vi "Test Executive.vi"(11 "Module Config":T30={"Name"="Test Executive", "Parent Q"=refnum, "Is Child?"=FALSE, "Index"=0, "Dirs"={"Root"=path "C:/MTE", "Config"=path "C:/MTE/Config", "Logs"=path "C:/MTE/Logs", "Reports"=path "C:/ATE/Reports", "App Data"=path "C:/ProgramData/Test Executive"}, "Simulate"=FALSE, "SimCtrl"=refnum}) -> ()   [LabVIEW 2018] (continued)
                    n1107 = List Folder(path=w2440) -> (filenames=w2441:string[], folder names=w2442:string[], error out=w2439:errorcluster)  [unwired: 3 in, 1 out]
                    n1108 = Array Size(array=w2441) -> (size(s)=w2443:i32)
                    n1109 = Array Size(array=w2442) -> (size(s)=w2444:i32)
                    n1110 = case shown="\"Passing\", \"PASS\"" w2449 {
                      tunnel: [_ "FAIL" "PASS" "ERROR" "ABORT"] -> w2448
                      frame "None", Default {
                      }
                      frame "Failing", "FAIL" {
                        (unwired) TRUE
                      }
                      frame "Passing", "PASS" {
                        (unwired) TRUE
                      }
                      frame "ERROR" {
                      }
                      frame "ABORT" {
                        (unwired) TRUE
                      }
                    }
                    n1111 = Format Into String(format string="%08d", w2437) -> (resulting string=w2435:string)  [unwired: 2 in, 1 out]
                    n1112 = Greater Than 0?(x=w2443) -> (x > 0?=w2446:bool)
                    n1113 = Greater Than 0?(x=w2444) -> (x > 0?=w2445:bool)
                    n1114 = local read "Seq Rslt"() -> (w2452:string)
                    n1115 = call <vilib>:"File.Check if File or Folder Exists.vi"("Path"=w2440) -> ("Exists"=w2447:bool)  [unwired: 6 in, 4 out]
                    n1116 = Or(x=w2446, y=w2445) -> (x .or. y?=w2438:bool)
                    n1117 = case shown="True" w2447 {
                      tunnel: w2453 -> [_ w2460]
                      tunnel: w2452 -> [_ w2459]
                      tunnel: w2450 -> [_ w2458]
                      tunnel: w2440 -> [_ w2457]
                      tunnel: w2448 -> [_ w2456]
                      tunnel: w2439 -> [_ _]
                      tunnel: w2438 -> [_ w2455]
                      tunnel: w2435 -> [_ w2454]
                      frame False {
                      }
                      frame True {
                        n1118 = case shown="True" w2455 {
                          tunnel: w2460 -> [_ w2472]
                          tunnel: w2459 -> [_ w2471]
                          tunnel: w2458 -> [_ w2466]
                          tunnel: w2457 -> [w2462 w2467]
                          tunnel: w2456 -> [_ w2470]
                          tunnel: [w2461 _] -> _
                          tunnel: w2454 -> [_ w2463]
                          frame False {
                            # "Folder is empty\nDelete it"
                            n1119 = Delete(path (use dialog)=w2462) -> (error out=w2461:errorcluster)  [unwired: 4 in, 2 out]
                          }
                          frame True {
                            # "Assign Task to Copy Folder"
                            n1120 = call "TestExec.Process Options for Archive UUT Folder.vi"("Sequence"=w2471, "Code"=w2463, "Result"=w2470, "Args"=w2472, "ArchiveDir"=w2466, "UUTDir"=w2467) -> ("Error"=w2468:errorcluster, "SubDirs"=w2464:string[], "New Name"=w2465:string)  [unwired: 2 in, 1 out]
                            n1121 = call "File.ArchiveMover, Assign Task.vi"("SubDirs"=w2464, "Q Name"="ArchiveMover", "error in"=w2468, "New Name"=w2465, "DestDir"=w2466, "Source"=w2467) -> ()  [unwired: 5 in, 1 out]
                          }
                        }
                      }
                    }
                  }
                  frame "ArchiveSummaryUUTData" {
                    n1122 = Unbundle By Name(w2489) -> ("UUT Dir"=w2480:path, "CfgFilePaths.Archive"=w2488:path)
                    n1123 = List Folder(path=w2480) -> (filenames=w2481:string[], folder names=w2482:string[], error out=w2479:errorcluster)  [unwired: 3 in, 1 out]
                    n1124 = Array Size(array=w2481) -> (size(s)=w2483:i32)
                    n1125 = Array Size(array=w2482) -> (size(s)=w2484:i32)
                    n1126 = Greater Than 0?(x=w2483) -> (x > 0?=w2486:bool)
                    n1127 = Greater Than 0?(x=w2484) -> (x > 0?=w2485:bool)
                    n1128 = call <vilib>:"File.Check if File or Folder Exists.vi"("Path"=w2480) -> ("Exists"=w2487:bool)  [unwired: 6 in, 4 out]
                    n1129 = Or(x=w2486, y=w2485) -> (x .or. y?=w2478:bool)
                    n1130 = case shown="True" w2487 {
                      tunnel: w2490 -> [_ w2495]
                      tunnel: w2488 -> [_ w2494]
                      tunnel: w2480 -> [_ w2493]
                      tunnel: w2479 -> [_ _]
                      tunnel: w2478 -> [_ w2492]
                      tunnel: [_ w2491] -> w2477
                      frame False {
                      }
                      frame True {
                        n1131 = case shown="True" w2492 {
                          tunnel: w2495 -> [_ w2511]
                          tunnel: w2494 -> [_ w2510]
                          tunnel: w2493 -> [w2497 w2509]
                          tunnel: [w2496 _] -> _
                          tunnel: [_ w2502] -> w2491
                          frame False {
                            # "Folder is empty\nDelete it"
                            n1132 = Delete(path (use dialog)=w2497) -> (error out=w2496:errorcluster)  [unwired: 4 in, 2 out]
                          }
                          frame True {
                            w2504 = T74 -5200 items=["No Error"=0, "Abort"=-2, "Misc"=-5000, "Fixture Error"=-5100, "File IO - General"=-5200, "FIle IO - Config Error"=-5201, "Instrument - General"=-5300, "Instrument - Serial Com"=-5301, "Instrument - Camera"=-5302, "Instrument - PS"=-5303, "Instrument - Oscilloscope"=-5304, "Instrument - Function Gen"=-5305, "Instrument - Load"=-5306, "Instrument - Meter"=-5307, "Instrument - Power Control"=-5308, "Instrument - Motion"=-5309, "Instrument - RF"=-5310, "System Exe"=-5400, "Image Processing"=-5500, "Communication"=-5600, "Script - Syntax Error"=-6000, "Script - Invalid Name or Param"=-6100, "Script - Timeout"=-6200, "Invalid Data"=-6300, "FW Update Error"=-6500] ("Std Code")
                            n1133 = call "TestExec.Process Options for Archive Summary UUT Folder.vi"("Args"=w2511, "ArchiveDir"=w2510, "UUTDir"=w2509) -> ("Destination Files"=w2505:path[], "Source Files"=w2508:path[], "Destination Path"=w2507:path)  [unwired: 5 in, 1 out]
                            n1134 = call <vilib>:"File.Create Folder if Does Not Exist.vi"("Path"=w2507) -> ("error out"=w2506:errorcluster, "Dup Path"=w2500:path)  [unwired: 8 in, 1 out]
                            n1135 = case shown="No Error" w2506 {
                              selector: w2506 -> [_ w2522]
                              tunnel: w2508 -> [w2515 _]
                              tunnel: w2505 -> [w2514 _]
                              tunnel: w2500 -> [_ _]
                              tunnel: [w2512 w2522] -> w2503
                              frame No Error {
                                n1136 = for {
                                tunnel: w2515 -> [w2521] mode=indexing
                                tunnel: [w2520] -> w2513 mode=indexing
                                tunnel: w2514 -> [w2517] mode=indexing
                                n1137 = Strip Path(path=w2517) -> (stripped path=w2519:path)  [unwired: 1 out]
                                n1138 = call <vilib>:"File.Create Folder if Does Not Exist.vi"("Path"=w2519) -> ("error out"=w2518:errorcluster)  [unwired: 8 in, 2 out]
                                n1139 = Copy(8:w2518, 9:TRUE ("overwrite (F)"), 10:w2517, 11:w2521) -> (0:w2520:errorcluster)  [unwired: 1 in, 2 out]
                                }
                                n1140 = Merge Errors(w2513) -> (w2512:errorcluster)
                              }
                              frame Error {
                              }
                            }
                            n1141 = Format Into String(format string="Error copying result summary files to: \"%s\".", w2500) -> (resulting string=w2499:string)  [unwired: 2 in, 1 out]
                            n1142 = call "Error.Set-Change Error Info.vi"("Std Code"=w2504, "Append Details"=FALSE, "error in"=w2503, "Description"=w2499) -> ("error out"=w2502:errorcluster)  [unwired: 7 in]
                          }
                        }
                      }
                    }
                  }
                  frame "ClientAttribute", "TestSetupAttribute" {
                    # "Cmd_ClientAttribute(Name,Value)"
                    n1143 = Unbundle By Name(w2526) -> ("RptHdr.Test Sequence.Config.Config_Item"=w2534:cluster{"Name":string, "Value":string}[])
                    n1144 = Index Array(array=w2527) -> (element #1=w2532:string, element #2=w2531:string)  [unwired: 2 in]
                    n1145 = call <vilib>:"Q.Enqueue Task.vi"("Top of Q"=TRUE, "Task Name"="Update Result Table", "Q In"=w2528) -> ()  [unwired: 7 in, 2 out]
                    n1146 = Bundle By Name(cluster=cluster{"Name":string, "Value":string} {"Name"="", "Value"=""} ("element"), "Name"=w2532, "Value"=w2531) -> (w2523:cluster{"Name":string, "Value":string})
                    n1147 = Build Array (concatenate)(w2534, w2523) -> (w2533:cluster{"Name":string, "Value":string}[])
                    n1148 = Bundle By Name(cluster=w2526, "RptHdr.Test Sequence.Config.Config_Item"=w2533) -> (w2525:T73)
                  }
                  frame "Comment" {
                    n1149 = Index Array(array=w2536) -> (element=w2539:string)  [unwired: 1 in]
                    n1150 = Unbundle By Name(w2537) -> ("Log"=w2540:refnum<class "Event Notification.lvclass">)
                    n1151 = call <vilib>:"Event Notification.Status Message.vi"("Display"=TRUE, "Log"=FALSE, "Level"=Event_Log.Log_Level."Normal", "Message"=w2539, "Event Notification in"=w2540) -> ()  [unwired: 7 in]
                  }
                  frame "CreateUUTFolder" {
                    n1152 = Unbundle By Name(w2558) -> ("CfgFilePaths.LocalData"=w2566:path)
                    n1153 = local read "SN"() -> (w2543:string)
                    n1154 = local read "Start Time"() -> (w2548:timestamp)
                    n1155 = call "File.Create UUT Dir.vi"("Start Time"=w2548, "SN"=w2543, "Local Data Dir"=w2566) -> ("error out"=w2565:errorcluster, "UUTDir"=w2552:path)  [unwired: 6 in, 1 out]
                    n1156 = Format Date/Time String(time format string (%c)="%Y%m%d_%H%M%S", seconds (now)=w2548) -> (date/time string=w2547:string)  [unwired: 1 in]
                    n1157 = Path To String(path=w2552) -> (string=w2568:string)
                    n1158 = Unbundle By Name(w2558) -> ("StaApp"=w2570:string)
                    n1159 = Build Array("SN", w2543) -> (w2546:string[])
                    n1160 = Build Array("UUTDir", w2568) -> (w2559:string[])
                    n1161 = Build Array("StartTime", w2547) -> (w2545:string[])
                    n1162 = To Variant(anything=w2552) -> (Variant=w2564:variant)
                    n1163 = Unbundle By Name(w2558) -> ("SeqMgr"=w2561:refnum<class "SeqMgr.lvclass">)
                    n1164 = Build Array(w2559, w2546, w2545) -> (w2563:string[][])
                    n1165 = call <vilib>:"Q.Enqueue Task.vi"("Data1"=w2564, "Q Name"=w2570, "Task Name"="Update UUT Folder") -> ()  [unwired: 7 in, 2 out]
                    n1166 = call <vilib>:"SeqMgr.Variables - Add, Replace.vi"("Name, Value"=w2563, "SeqMgr in"=w2561) -> ("SeqMgr out"=w2562:refnum<class "SeqMgr.lvclass">)  [unwired: 8 in, 1 out]
                    n1167 = Bundle By Name(cluster=w2558, "SeqMgr"=w2562, "UUT Dir"=w2552) -> (w2560:T73)
                    n1168 = Unbundle By Name(w2551) -> ("Log"=w2556:refnum<class "Event Notification.lvclass">)
                    n1169 = Format Into String(format string="Create UUT Folder \"%s\"", w2552) -> (resulting string=w2557:string)  [unwired: 2 in, 1 out]
                    n1170 = call <vilib>:"Event Notification.Status Message.vi"("Log"=TRUE, "Level"=Event_Log.Log_Level."Debug1", "Message"=w2557, "Event Notification in"=w2556) -> ()  [unwired: 8 in]
                  }
                  frame "CreateCsvReport" {
                    # "Cmd_CreateCsvReport(Folder)"
                    n1171 = Unbundle By Name(w2581) -> ("RptHdr"=w2589:T70, "RptUUT"=w2605:T50, "Data.Meas"=w2604:T38[], "ResultState"=w2598:T63)
                    n1172 = local read "Comment"() -> (w2582:string)
                    n1173 = Unbundle By Name(w2598) -> ("Code"=w2597:i32, "Description"=w2596:string, "State"=w2595:T1)
                    n1174 = Index Array(array=w2585) -> (element=w2592:string)  [unwired: 1 in]
                    n1175 = case shown="True" "Comment At End" {
                      tunnel: w2582 -> [w2607 w2612]
                      tunnel: [w2607 w2611] -> w2580
                      tunnel: w2581 -> [w2606 w2610]
                      tunnel: [w2606 w2609] -> w2579
                      frame False {
                      }
                      frame True {
                        n1176 = Bundle By Name(cluster=w2610, "Lists.CmtPrmpt"=TRUE) -> (w2609:T73)
                        n1177 = call "TestExec.Prompt for entering Comment.vi"("Comment"=w2612) -> ("Comment Out"=w2611:string)  [unwired: 10 in]
                      }
                    }
                    n1178 = case shown="\"Passing\", \"PASS\"" w2595 {
                      tunnel: [TestResult.Symptom.State."Completed" ("Result.Result") TestResult.Symptom.State."Pass" ("Result.Result") TestResult.Symptom.State."Fail" ("Result.Result") TestResult.Symptom.State."Aborted" ("Result.Result") TestResult.Symptom.State."Error" ("Result.Result")] -> w2594
                      frame "None", Default {
                      }
                      frame "Passing", "PASS" {
                      }
                      frame "Failing", "FAIL" {
                      }
                      frame "ABORT" {
                      }
                      frame "ERROR" {
                      }
                    }
                    n1179 = String To Path(string=w2592) -> (path=w2591:path)
                    n1180 = Bundle By Name(cluster=w2605, "Measurements.Measurement"=w2604, "Result.Code"=w2597, "Result.Description"=w2596, "Result.Result"=w2594) -> (w2600:T50)
                    n1181 = local read "Duration(s)"() -> (w2587:dbl)
                    n1182 = call <vilib>:"File.Check if File or Folder Exists.vi"("Path"=w2591) -> ("Exists"=w2590:bool, "Dup Path"=w2571:path)  [unwired: 6 in, 3 out]
                    n1183 = Bundle By Name(cluster=w2589, "Test Run.Comment"=w2580, "Test Run.Duration(s)"=w2587) -> (w2588:T70)
                    n1184 = Unbundle By Name(w2588) -> ("Station"=w2603:T47, "Test Run"=w2602:T48, "Test Sequence"=w2601:T49)
                    n1185 = Bundle By Name(cluster=w2579, "RptHdr.Test Run.Comment"=w2580) -> (w2578:T73)
                    n1186 = Build Array(w2600) -> (w2599:T50[])
                    n1187 = Bundle By Name(cluster=T46 {"#attributes"={"Version"="MTE_1.0.0"}, "Station"={"Name"="", "PN"="", "SN"="", "Rev"="", "PC Name"="", "Location"="", "HW_Config"={"HW_Item"=[]}, "SW_Config"={"SW_Item"=[]}}, "Test Run"={"Operator"="", "Start Time"=timestamp(0 s since 1904-01-01), "Duration(s)"=0.0, "Mode"="", "Comment"="", "ProcessStep"=""}, "Test Sequence"={"Name"="", "Config"={"Config_Item"=[]}}, "UUTs"={"UUT"=[]}} ("Test Result"), "Station"=w2603, "Test Run"=w2602, "Test Sequence"=w2601, "UUTs.UUT"=w2599) -> (w2593:T46)
                    n1188 = case shown="False" w2590 {
                      tunnel: w2593 -> [_ w2622]
                      tunnel: w2571 -> [w2617 w2620]
                      tunnel: [w2615 w2621] -> w2584
                      frame False {
                        w2616 = T74 -6100 items=["No Error"=0, "Abort"=-2, "Misc"=-5000, "Fixture Error"=-5100, "File IO - General"=-5200, "FIle IO - Config Error"=-5201, "Instrument - General"=-5300, "Instrument - Serial Com"=-5301, "Instrument - Camera"=-5302, "Instrument - PS"=-5303, "Instrument - Oscilloscope"=-5304, "Instrument - Function Gen"=-5305, "Instrument - Load"=-5306, "Instrument - Meter"=-5307, "Instrument - Power Control"=-5308, "Instrument - Motion"=-5309, "Instrument - RF"=-5310, "System Exe"=-5400, "Image Processing"=-5500, "Communication"=-5600, "Script - Syntax Error"=-6000, "Script - Invalid Name or Param"=-6100, "Script - Timeout"=-6200, "Invalid Data"=-6300, "FW Update Error"=-6500] ("Std Code")
                        n1189 = Format Into String(format string="Can not create CSV report.  Dir does not exist: \"%s\"", w2617) -> (resulting string=w2614:string)  [unwired: 2 in, 1 out]
                        n1190 = call "Error.Set-Change Error Info.vi"("Std Code"=w2616, "Description"=w2614, "Set Error"=TRUE) -> ("error out"=w2615:errorcluster)  [unwired: 8 in]
                      }
                      frame True {
                        n1191 = call "Result.Report Creator.vi"("Use UUTFolderName"=TRUE, "Data"=w2622, "Format"=Result.Report_Format_Selector."CSV", "OutputDir"=w2620) -> ("error out"=w2621:errorcluster)  [unwired: 6 in, 1 out]
                      }
                    }
                    n1192 = Unbundle By Name(w2572) -> ("Log"=w2576:refnum<class "Event Notification.lvclass">)
                    n1193 = Format Into String(format string="Create CSV Report in \"%s\"", w2571) -> (resulting string=w2577:string)  [unwired: 2 in, 1 out]
                    n1194 = call <vilib>:"Event Notification.Status Message.vi"("Log"=TRUE, "Level"=Event_Log.Log_Level."Debug1", "Message"=w2577, "Event Notification in"=w2576) -> ()  [unwired: 8 in]
                  }
                  frame "DataPrompt" {
                    # "DataPrompt(PromptText,VarName)"
                    n1195 = while {
                      shift-right: [w2638] -> w2632
                      shift-left: w2633 -> [w2641]
                      shift-right: [w2637] -> _
                      shift-left: "Init" -> [w2642]
                      tunnel: w2631 -> [w2640]
                      tunnel: w2630 -> [w2639]
                      tunnel: [w2635] -> w2629
                      stop <- w2636 stop-if-true
                      n1196 = case shown="\"Done\", Default" w2642 {
                        tunnel: w2641 -> [w2647 w2663 w2677 w2703 w2710 w2714]
                        tunnel: w2640 -> [w2643 w2660 _ w2701 _ _]
                        tunnel: w2639 -> [w2645 _ _ _ _ w2717]
                        tunnel: [w2647 w2663 w2677 w2704 w2710 w2714] -> w2638
                        tunnel: [w2646 "Wait on Input" "Read Data" "Disable Controls" "Done" _] -> w2637
                        tunnel: [_ _ _ _ _ TRUE] -> w2636
                        tunnel: [w2644 _ _ _ _ w2717] -> w2635
                        frame "Init" {
                          n1197 = case shown="No Error" w2645 {
                            selector: w2645 -> [_ w2655]
                            tunnel: ["Enable Controls" "Done"] -> w2646
                            tunnel: [_ w2655] -> w2644
                            tunnel: w2643 -> [w2650 _]
                            frame No Error {
                              w2648 = T6."Prompt" ("Test Status Tab")
                              n1198 = Index Array(array=w2650) -> (element=→"OperPrompt2":string)  [unwired: 1 in]
                              n1199 = local write "Test Status Tab"(w2648) -> ()
                              n1200 = local write "Test Status Tab Sel"(w2648) -> ()
                              n1201 = property on="Status" class="Str"("Text.Text"="Waiting for Operator input on Prompt page.", "Text.BGColor"=u32 16774001, "Blinking"=TRUE) -> ()  [unwired: 2 in, 2 out]
                            }
                            frame Error {
                            }
                          }
                        }
                        frame "Enable Controls" {
                          w2661 = T36."Enabled" ("Disabled")
                          n1202 = Index Array(array=w2660, index=2) -> (element=w2657:string)
                          n1203 = property on="Prompt2_OK" class="Bool"("DisabledEnum"=w2661) -> ()  [unwired: 2 in, 2 out]
                          n1204 = property on="Prompt YES" class="Bool"("DisabledEnum"=w2661) -> ()  [unwired: 2 in, 2 out]
                          n1205 = property on="Prompt NO" class="Bool"("DisabledEnum"=w2661) -> ()  [unwired: 2 in, 2 out]
                          n1206 = property on="OperInput Data" class="Str"("DisabledEnum"=w2661) -> (error out=w2658:errorcluster)  [unwired: 2 in, 1 out]
                          n1207 = case shown="\"\", \"0\", Default" w2657 {
                            tunnel: w2658 -> [_ _ _]
                            frame "", "0", Default {
                              w2665 = FALSE ("Visible")
                              n1208 = property on="Prompt2_OK" class="Bool"("Visible"=TRUE) -> ()  [unwired: 2 in, 2 out]
                              n1209 = property on="OperInput Data" class="Str"("Visible"=TRUE ("Key Focus")) -> ()  [unwired: 2 in, 2 out]
                              n1210 = property on="Prompt YES" class="Bool"("Visible"=w2665) -> ()  [unwired: 2 in, 2 out]
                              n1211 = property on="Prompt NO" class="Bool"("Visible"=w2665) -> ()  [unwired: 2 in, 2 out]
                              n1212 = property on="OperInput Data" class="Str"("Key Focus"=TRUE) -> ()  [unwired: 2 in, 2 out]
                            }
                            frame "1" {
                              w2670 = FALSE ("Visible")
                              n1213 = property on="OperInput Data" class="Str"("Visible"=FALSE) -> ()  [unwired: 2 in, 2 out]
                              n1214 = property on="Prompt YES" class="Bool"("Visible"=w2670) -> ()  [unwired: 2 in, 2 out]
                              n1215 = property on="Prompt NO" class="Bool"("Visible"=w2670) -> ()  [unwired: 2 in, 2 out]
                              n1216 = property on="Prompt2_OK" class="Bool"("Key Focus"=TRUE) -> ()  [unwired: 2 in, 2 out]
                              n1217 = property on="Prompt2_OK" class="Bool"("Visible"=TRUE ("Key Focus")) -> ()  [unwired: 2 in, 2 out]
                            }
                            frame "2" {
                              w2673 = TRUE ("Visible")
                              n1218 = property on="OperInput Data" class="Str"("Visible"=FALSE) -> ()  [unwired: 2 in, 2 out]
                              n1219 = property on="Prompt2_OK" class="Bool"("Visible"=FALSE ("Key Focus")) -> ()  [unwired: 2 in, 2 out]
                              n1220 = property on="Prompt YES" class="Bool"("Visible"=w2673) -> ()  [unwired: 2 in, 2 out]
                              n1221 = property on="Prompt NO" class="Bool"("Visible"=w2673) -> ()  [unwired: 2 in, 2 out]
                              n1222 = property on="Prompt YES" class="Bool"("Key Focus"=TRUE ("Visible")) -> ()  [unwired: 2 in, 2 out]
                            }
                          }
                        }
                        frame "Wait on Input" {
                          n1223 = while {
                            stop <- w2678 stop-if-true
                            n1224 = event shown="[1] \"Prompt2_OK\": Value Change" {
                              selector: _ -> [_ _ _ _]
                              dyn-events: _ -> [_ _ _ _]
                              timeout: 100 -> [_ _ _ _]
                              tunnel: [w2680 TRUE TRUE TRUE] -> w2678
                              event Timeout {
                                n1225 = event-data() -> ()  [unwired: 1 in, 3 out]
                                n1226 = local read "Abort Flag"() -> (w2680:bool)
                              }
                              event "Prompt2_OK": Value Change {
                                n1227 = event-data() -> ()  [unwired: 1 in, 6 out]
                              }
                              event "Prompt YES", "Prompt NO": Value Change {
                                n1228 = event-data() -> ()  [unwired: 1 in, 6 out]
                                n1229 = Select(t="YES", s="Prompt YES", f="NO") -> (s? t:f=w2683:string)
                                n1230 = local write "OperInput Data"(w2683) -> ()
                              }
                              event "OperInput Data": Value Change {
                                n1231 = event-data() -> ()  [unwired: 1 in, 6 out]
                              }
                            }
                          }
                        }
                        frame "Read Data" {
                          n1232 = Index Array(array=w2701, index=1) -> (element=w2697:string)
                          n1233 = call <vilib>:"Trim Whitespace.vi"("string"=w2697) -> ("trimmed string"=w2696:string)  [unwired: 1 in]
                          n1234 = call <vilib>:"Trim Whitespace.vi"("string"="OperInput Data") -> ("trimmed string"=w2688:string)  [unwired: 1 in]
                          n1235 = Empty String/Path?(string/path=w2696) -> (empty?=w2699:bool)
                          n1236 = Select(t="OperatorDataInput", s=w2699, f=w2696) -> (s? t:f=w2694:string)
                          n1237 = Build Array(w2694, w2688) -> (w2695:string[])
                          n1238 = Unbundle By Name(w2703) -> ("SeqMgr"=w2706:refnum<class "SeqMgr.lvclass">)
                          n1239 = Build Array(w2695) -> (w2702:string[][])
                          n1240 = Format Into String(format string="Input data = %s", w2688) -> (resulting string=w2692:string)  [unwired: 2 in, 1 out]
                          n1241 = call <vilib>:"SeqMgr.Variables - Add, Replace.vi"("Name, Value"=w2702, "SeqMgr in"=w2706) -> ("SeqMgr out"=w2705:refnum<class "SeqMgr.lvclass">)  [unwired: 8 in, 1 out]
                          n1242 = Bundle By Name(cluster=w2703, "SeqMgr"=w2705) -> (w2704:T73)
                          n1243 = property on="Status" class="Str"("Text.Text"=w2692, "Text.BGColor"=u32 16448250, "Blinking"=FALSE) -> ()  [unwired: 2 in, 2 out]
                        }
                        frame "Disable Controls" {
                          w2708 = T36."Disabled and Grayed Out" ("Disabled")
                          n1244 = property on="Prompt2_OK" class="Bool"("DisabledEnum"=w2708) -> ()  [unwired: 2 in, 2 out]
                          n1245 = property on="Prompt YES" class="Bool"("DisabledEnum"=w2708) -> ()  [unwired: 2 in, 2 out]
                          n1246 = property on="Prompt NO" class="Bool"("DisabledEnum"=w2708) -> ()  [unwired: 2 in, 2 out]
                          n1247 = property on="OperInput Data" class="Str"("DisabledEnum"=w2708) -> ()  [unwired: 2 in, 2 out]
                        }
                        frame "Done", Default {
                          n1248 = Unbundle By Name(w2714) -> ("Opts.DispDetails"=w2715:bool)
                          n1249 = invoke on="OperPrompt2" class="Str" method="Reinit To Default"() -> ()  [unwired: 3 in, 3 out]
                          n1250 = invoke on="OperInput Data" class="Str" method="Reinit To Default"() -> ()  [unwired: 3 in, 3 out]
                          n1251 = Select(t=1, s=w2715, f=0) -> (s? t:f=w2711:i32)
                          n1252 = property on="Prompt2_OK" class="Bool"("DisabledEnum"=T36."Disabled and Grayed Out" ("Disabled")) -> ()  [unwired: 2 in, 2 out]
                          n1253 = local write "Test Status Tab Sel"(w2711) -> ()
                          n1254 = local write "Test Status Tab"(w2711) -> ()
                        }
                      }
                    }
                  }
                  frame "Delay", "Wait" {
                    # "Wait(Secs)"
                    n1255 = Unbundle By Name(w2731) -> ("Log"=w2720:refnum<class "Event Notification.lvclass">)
                    n1256 = local read "Status"() -> (w2728:string)
                    n1257 = Index Array(array=w2719) -> (element=w2729:string)  [unwired: 1 in]
                    n1258 = Concatenate Strings(w2728, "\r\n") -> (w2727:string)
                    n1259 = Fract/Exp String To Number(string=w2729) -> (number=w2726:dbl)  [unwired: 3 in, 1 out]
                    n1260 = Format Into String(format string="Delaying for %s seconds.", initial string=w2727, w2729) -> (resulting string=w2725:string)  [unwired: 1 in, 1 out]
                    n1261 = call <vilib>:"Event Notification.Status Message.vi"("Log"=FALSE, "Level"=Event_Log.Log_Level."Normal", "Message"=w2725, "Event Notification in"=w2720) -> ()  [unwired: 8 in]
                    n1262 = call <vilib>:"High Resolution Relative Seconds.vi"() -> ("relative seconds"=w2730:dbl)
                    n1263 = while {
                      tunnel: w2730 -> [w2745]
                      tunnel: w2726 -> [w2739]
                      stop <- w2743 stop-if-true
                      # "Remain"
                      # "Elapsed"
                      n1264 = call <vilib>:"High Resolution Relative Seconds.vi"() -> ("relative seconds"=w2746:dbl)
                      n1265 = Subtract(x=w2746, y=w2745) -> (x-y=w2738:dbl)
                      n1266 = Subtract(x=w2739, y=w2738) -> (x-y=w2736:dbl)
                      n1267 = local read "Status"() -> (w2742:string)
                      n1268 = Less Or Equal To 0?(x=w2736) -> (x <= 0?=w2737:bool)
                      n1269 = Multiply(x=w2736, y=1000.0) -> (x*y=w2733:dbl)
                      n1270 = local read "Abort Flag"() -> (w2744:bool)
                      n1271 = Concatenate Strings(w2742, " .") -> (w2740:string)
                      n1272 = To Unsigned Long Integer(number=w2733) -> (unsigned 32bit integer=w2734:u32)
                      n1273 = local write "Status"(w2740) -> ()
                      n1274 = case shown="False" w2737 {
                        tunnel: w2734 -> [w2750 _]
                        frame False {
                          n1275 = In Range and Coerce(upper limit=u32 500 ("lower limit"), x=w2750, lower limit=u32 10) -> (coerced(x)=w2747:u32)  [unwired: 1 out]
                          n1276 = Wait (ms)(milliseconds to wait=w2747) -> ()  [unwired: 1 out]
                        }
                        frame True {
                        }
                      }
                      n1277 = Or(x=w2737, y=w2744) -> (x .or. y?=w2743:bool)
                    }
                  }
                  frame "DeviceEnumCheck" {
                    # "EnumCheck(VID,PID,[RtnVarName])"
                    n1278 = Index Array(array=w2756) -> (element #1=w2755:string, element #2=w2754:string, element #3=w2760:string)  [unwired: 3 in]
                    n1279 = case shown="\"\"" w2760 {
                      selector: w2760 -> [w2783 _]
                      tunnel: [w2783 "DeviceIsEnumerated"] -> w2759
                      frame Default {
                      }
                      frame "" {
                      }
                    }
                    n1280 = Empty String/Path?(string/path=w2755) -> (empty?=w2753:bool)
                    n1281 = Empty String/Path?(string/path=w2754) -> (empty?=w2752:bool)
                    n1282 = And(x=w2753, y=w2752) -> (x .and. y?=w2751:bool)
                    n1283 = case shown="True" w2751 {
                      tunnel: w2759 -> [w2768 _]
                      tunnel: w2758 -> [w2766 w2778]
                      tunnel: [w2765 w2776] -> w2757
                      tunnel: w2755 -> [w2762 _]
                      tunnel: w2754 -> [w2761 _]
                      frame False {
                        n1284 = call "USB.Check Device using PID and VID.vi"("PID"=w2761, "VID"=w2762) -> ("error out"=w2763:errorcluster, "Found"=w2764:bool)  [unwired: 6 in, 2 out]
                        n1285 = call <vilib>:"Clear Errors.vi"("error in (no error)"=w2763) -> ()  [unwired: 5 in, 2 out]
                        n1286 = Select(t="1", s=w2764, f="0") -> (s? t:f=w2770:string)
                        n1287 = Build Array(w2768, w2770) -> (w2769:string[])
                        n1288 = Unbundle By Name(w2766) -> ("SeqMgr"=w2774:refnum<class "SeqMgr.lvclass">)
                        n1289 = Build Array(w2769) -> (w2767:string[][])
                        n1290 = call <vilib>:"SeqMgr.Variables - Add, Replace.vi"("Name, Value"=w2767, "SeqMgr in"=w2774) -> ("SeqMgr out"=w2773:refnum<class "SeqMgr.lvclass">)  [unwired: 8 in, 1 out]
                        n1291 = Bundle By Name(cluster=w2766, "SeqMgr"=w2773) -> (w2765:T73)
                      }
                      frame True {
                        w2775 = T74 -6100 items=["No Error"=0, "Abort"=-2, "Misc"=-5000, "Fixture Error"=-5100, "File IO - General"=-5200, "FIle IO - Config Error"=-5201, "Instrument - General"=-5300, "Instrument - Serial Com"=-5301, "Instrument - Camera"=-5302, "Instrument - PS"=-5303, "Instrument - Oscilloscope"=-5304, "Instrument - Function Gen"=-5305, "Instrument - Load"=-5306, "Instrument - Meter"=-5307, "Instrument - Power Control"=-5308, "Instrument - Motion"=-5309, "Instrument - RF"=-5310, "System Exe"=-5400, "Image Processing"=-5500, "Communication"=-5600, "Script - Syntax Error"=-6000, "Script - Invalid Name or Param"=-6100, "Script - Timeout"=-6200, "Invalid Data"=-6300, "FW Update Error"=-6500] ("Code")
                        n1292 = Unbundle By Name(w2778) -> ("Lists.Limits"=w2782:variant, "ResultState"=w2781:T63)
                        n1293 = call "TestExec.Set Result State.vi"("Code Enum"=w2775, "Limits"=w2782, "Description"="DeviceEnumCheck Error, both VID and PID arguements cannot be empty.", "State"=SeqMgr.Result_State_Enum."ERROR", "Result State In"=w2781) -> ("Result State Out"=w2777:T63)  [unwired: 6 in]
                        n1294 = Bundle By Name(cluster=w2778, "ResultState"=w2777) -> (w2776:T73)
                      }
                    }
                  }
                  frame "Devcon_ListDevices", "Devcon_RemoveDevice", "Devcon_RemoveDevices", "Devcon_Rescan" {
                    n1295 = Unbundle By Name(w2788) -> ("CfgFilePaths.Devcon"=w2791:path)
                    n1296 = case shown="\"Devcon_RemoveDevices\"" w2793 {
                      tunnel: w2792 -> [_ w2806 w2823 w2844 _]
                      tunnel: w2791 -> [_ w2807 w2824 w2845 w2860]
                      tunnel: [_ w2795 w2821 w2838 w2852] -> w2786
                      tunnel: [_ w2794 w2814 w2828 w2853] -> w2785
                      frame Default {
                      }
                      frame "Devcon_ListDevices" {
                        n1297 = Index Array(array=w2806) -> (element #1=w2805:string, element #2=w2804:string)  [unwired: 2 in]
                        n1298 = Equal?(x=w2804, y="1") -> (x = y?=w2802:bool)
                        n1299 = call "Devcon.Find Devices.vi"("State(Present(F), All(T))"=w2802, "DeviceID"=w2805, "DevconEXE"=w2807) -> ("error out"=w2794:errorcluster, "Device List"=w2798:string[][], "Device Cnt"=w2800:i32)  [unwired: 4 in, 2 out]
                        n1300 = for {
                          tunnel: w2798 -> [w2813] mode=indexing
                          tunnel: [w2808] -> w2796 mode=indexing
                          i -> [w2811]
                          n1301 = Index Array(array=w2813) -> (element=w2809:string)  [unwired: 1 in]
                          n1302 = Format Into String(format string="Device_%d", w2811) -> (resulting string=w2810:string)  [unwired: 2 in, 1 out]
                          n1303 = Build Array(w2810, w2809) -> (w2808:string[])
                        }
                        n1304 = Number To Decimal String(number=w2800) -> (decimal integer string=w2799:string)  [unwired: 1 in]
                        n1305 = Build Array("DeviceCount", w2799) -> (w2797:string[])
                        n1306 = Build Array (concatenate)(w2797, w2796) -> (w2795:string[][])
                      }
                      frame "Devcon_RemoveDevice" {
                        n1307 = Index Array(array=w2823) -> (element #1=w2822:string)  [unwired: 2 in, 1 out]
                        n1308 = call "Devcon.Remove Device.vi"("DeviceID"=w2822, "DevconEXE"=w2824) -> ("error out"=w2814:errorcluster, "Success"=w2817:bool)  [unwired: 6 in, 2 out]
                        n1309 = Select(t="1", s=w2817, f="0") -> (s? t:f=w2819:string)
                        n1310 = Build Array("DeviceRemoveSuccess", w2819) -> (w2816:string[])
                        n1311 = Build Array(w2816) -> (w2821:string[][])
                      }
                      frame "Devcon_RemoveDevices" {
                        n1312 = Index Array(array=w2844) -> (element #1=w2843:string, element #2=w2826:string)  [unwired: 2 in]
                        n1313 = Equal?(x=w2826, y="1") -> (x = y?=w2825:bool)
                        n1314 = call "Devcon.Remove Devices.vi"("State(Present(F), All(T))"=w2825, "DeviceID"=w2843, "DevconEXE"=w2845) -> ("error out"=w2828:errorcluster, "Success"=w2833:bool, "Device List"=w2836:string[][])  [unwired: 4 in, 2 out]
                        n1315 = Array Size(array=w2836) -> (size(s)=w2837:i32[])
                        n1316 = Index Array(array=w2837) -> (element=w2835:i32)  [unwired: 1 in]
                        n1317 = for {
                          tunnel: w2836 -> [w2851] mode=indexing
                          tunnel: [w2846] -> w2839 mode=indexing
                          i -> [w2849]
                          n1318 = Index Array(array=w2851) -> (element=w2847:string)  [unwired: 1 in]
                          n1319 = Format Into String(format string="Device_%d", w2849) -> (resulting string=w2848:string)  [unwired: 2 in, 1 out]
                          n1320 = Build Array(w2848, w2847) -> (w2846:string[])
                        }
                        n1321 = Select(t="1", s=w2833, f="0") -> (s? t:f=w2831:string)
                        n1322 = Number To Decimal String(number=w2835) -> (decimal integer string=w2841:string)  [unwired: 1 in]
                        n1323 = Build Array("DeviceCount", w2841) -> (w2840:string[])
                        n1324 = Build Array("DeviceRemoveSuccess", w2831) -> (w2829:string[])
                        n1325 = Build Array (concatenate)(w2840, w2839, w2829) -> (w2838:string[][])
                      }
                      frame "Devcon_Rescan" {
                        n1326 = call "Devcon.Rescan for New Devices.vi"("DevconEXE"=w2860) -> ("error out"=w2853:errorcluster, "Success"=w2854:bool)  [unwired: 9 in]
                        n1327 = Select(t="1", s=w2854, f="0") -> (s? t:f=w2858:string)
                        n1328 = Build Array("DeviceRescanSuccess", w2858) -> (w2856:string[])
                        n1329 = Build Array(w2856) -> (w2852:string[][])
                      }
                    }
                    n1330 = Unbundle By Name(w2788) -> ("SeqMgr"=w2790:refnum<class "SeqMgr.lvclass">)
                    n1331 = call <vilib>:"SeqMgr.Variables - Add, Replace.vi"("Name, Value"=w2786, "SeqMgr in"=w2790) -> ("SeqMgr out"=w2789:refnum<class "SeqMgr.lvclass">)  [unwired: 8 in, 1 out]
                    n1332 = Bundle By Name(cluster=w2788, "SeqMgr"=w2789) -> (w2787:T73)
                  }
                  frame "Error", "SetError" {
                    # "SetError(Code, Desc)"
                    n1333 = Index Array(array=w2873) -> (element #1=w2862:string, element #2=w2866:string)  [unwired: 2 in]
                    n1334 = Unbundle By Name(w2871) -> ("Lists.Limits"=w2878:variant)
                    n1335 = Decimal String To Number(string=w2862) -> (number=w2864:i32)  [unwired: 2 in, 1 out]
                    n1336 = Get Variant Attribute(Variant=w2878, name="CodePrefix", default value (empty Variant)=T25 {"Name"="", "LimType"=enum."None", "LL"="", "UL"="", "Units"="", "FailCode"=0, "FailDesc"=""} ("Result.Test Limit Item")) -> (value=w2880:T25)  [unwired: 1 in, 3 out]
                    n1337 = Equal To 0?(x=w2864) -> (x = 0?=w2865:bool)
                    n1338 = Unbundle By Name(w2880) -> ("FailCode"=w2876:i32)
                    n1339 = Select(t=-5000, s=w2865, f=w2864) -> (s? t:f=w2861:i32)
                    n1340 = call <vilib>:"Q.Enqueue Task.vi"("Top of Q"=TRUE, "Task Name"="Sta Test Status", "Q In"=w2868) -> ()  [unwired: 7 in, 2 out]
                    n1341 = call "TestExec.Append Fault Code Prefix.vi"("Positive(F)\\Negative(T)"=TRUE ("Positive(F)\\Negative(T)"), "FaultCode"=w2861, "FaultCode Prefix"=w2876) -> ("New Fault Code"=w2875:i32)  [unwired: 8 in]
                    n1342 = Bundle By Name(cluster=w2871, "ResultState.State"=SeqMgr.Result_State_Enum."ERROR" ("State"), "ResultState.Code"=w2875, "ResultState.Description"=w2866) -> (w2874:T73)
                    n1343 = Format Into String(format string="Error set by sequence: %s", w2866) -> (resulting string=w2867:string)  [unwired: 2 in, 1 out]
                    n1344 = Unbundle By Name(w2874) -> ("SeqMgr"=w2890:refnum<class "SeqMgr.lvclass">)
                    n1345 = Unbundle By Name(w2872) -> ("Log"=w2884:refnum<class "Event Notification.lvclass">)
                    n1346 = call <vilib>:"SeqMgr.Variables - Add, Replace.vi"("Name, Value"=string[][] [["Error", "1"]] ("appended array"), "SeqMgr in"=w2890) -> ("SeqMgr out"=w2889:refnum<class "SeqMgr.lvclass">)  [unwired: 8 in, 1 out]
                    n1347 = Bundle By Name(cluster=w2874, "SeqMgr"=w2889) -> (w2887:T73)
                    n1348 = call <vilib>:"Event Notification.Status Message.vi"("Log"=TRUE, "Level"=Event_Log.Log_Level."Verbose", "Message"=w2867, "Event Notification in"=w2884) -> ()  [unwired: 8 in]
                  }
                  frame "ImagePrompt" {
                    # "ImagePrompt(PromptMessage,ImageFileFolder,ImageFileName,[ResultAttributeName])"
                    n1349 = while {
                      shift-right: [w2907] -> w2896
                      shift-left: w2897 -> [w2908]
                      tunnel: w2895 -> [_]
                      shift-right: [w2900] -> _
                      shift-left: "Init" -> [w2909]
                      shift-right: [w2901] -> _
                      shift-left: w2893 -> [w2905]
                      shift-right: [w2903] -> _
                      shift-left: _ -> [w2904]
                      tunnel: w2892 -> [w2902]
                      tunnel: w2891 -> [w2898]
                      stop <- w2906 stop-if-true
                      n1350 = case shown="\"Load Image\"" w2909 {
                        tunnel: w2908 -> [w2932 w2952 w2960 w3014]
                        tunnel: [w2932 w2952 w2960 w3014] -> w2907
                        tunnel: ["Load Image" "Get Input" "Done" "Done"] -> w2899
                        tunnel: [_ _ _ TRUE] -> w2906
                        tunnel: w2905 -> [_ _ _ w3001]
                        tunnel: [w2914 w2948 w2954 w3001] -> w2901
                        tunnel: w2904 -> [_ w2947 w2959 w2999]
                        tunnel: [w2923 w2947 w2958 w2999] -> w2903
                        tunnel: w2902 -> [w2928 _ _ _]
                        tunnel: w2898 -> [_ _ _ w2996]
                        frame "Init" {
                          w2919 = FALSE  # OK
                          w2920 = FALSE  # Timeout
                          w2929 = path ""  # Image
                          w2930 = ""  # Name
                          w2912 = T36."Enabled" ("Disabled")
                          n1351 = Index Array(array=w2928) -> (element #1=→"OperPrompt":string, element #2=w2922:string, element #3=w2921:string, element #4=w2926:string)  [unwired: 4 in]
                          n1352 = call "TestExec.Script Function Params to Path.vi"("File"=w2921, "Folder"=w2922) -> ("error out"=w2913:errorcluster, "Exists"=w2917:bool, "Path"=w2915:path)  [unwired: 7 in]
                          n1353 = case shown="\"\"" w2926 {
                            selector: w2926 -> [w2940 _]
                            tunnel: [w2940 "Operator Image Prompt"] -> w2925
                            frame Default {
                            }
                            frame "" {
                            }
                          }
                          n1354 = Not(x=w2917) -> (.not. x?=w2916:bool)
                          n1355 = Or(x=w2916, y=w2913) -> (x .or. y?=w2918:bool)
                          n1356 = case shown="True" w2918 {
                            tunnel: w2915 -> [_ w2934]
                            tunnel: [_ w2933] -> w2914
                            frame False {
                            }
                            frame True {
                              w2939 = T74 -5200 items=["No Error"=0, "Abort"=-2, "Misc"=-5000, "Fixture Error"=-5100, "File IO - General"=-5200, "FIle IO - Config Error"=-5201, "Instrument - General"=-5300, "Instrument - Serial Com"=-5301, "Instrument - Camera"=-5302, "Instrument - PS"=-5303, "Instrument - Oscilloscope"=-5304, "Instrument - Function Gen"=-5305, "Instrument - Load"=-5306, "Instrument - Meter"=-5307, "Instrument - Power Control"=-5308, "Instrument - Motion"=-5309, "Instrument - RF"=-5310, "System Exe"=-5400, "Image Processing"=-5500, "Communication"=-5600, "Script - Syntax Error"=-6000, "Script - Invalid Name or Param"=-6100, "Script - Timeout"=-6200, "Invalid Data"=-6300, "FW Update Error"=-6500] ("Std Code")
                              n1357 = Path To String(path=w2934) -> (string=w2937:string)
                              n1358 = Format Into String(format string="Image file does not exist: \"%s\".", w2937) -> (resulting string=w2936:string)  [unwired: 2 in, 1 out]
                              n1359 = call "Error.Set-Change Error Info.vi"("Std Code"=w2939, "Description"=w2936, "Set Error"=TRUE) -> ("error out"=w2933:errorcluster)  [unwired: 8 in]
                            }
                          }
                          n1360 = Bundle("Name"=w2930, "Image"=w2929, "Timeout"=w2920, "OK"=w2919) -> (w2924:T79)  [unwired: 1 in]
                          n1361 = Bundle By Name(cluster=w2924, "Name"=w2925, "Image"=w2915) -> (w2923:T79)
                          n1362 = invoke on="OperPict" class="Pict" method="Reinit To Default"() -> ()  [unwired: 3 in, 3 out]
                          n1363 = property on="Open Image File" class="Bool"("DisabledEnum"=w2912) -> ()  [unwired: 2 in, 2 out]
                          n1364 = property on="OperNo" class="Bool"("DisabledEnum"=w2912) -> ()  [unwired: 2 in, 2 out]
                          n1365 = property on="OperOK" class="Bool"("DisabledEnum"=w2912) -> ()  [unwired: 2 in, 2 out]
                        }
                        frame "Load Image" {
                          n1366 = Unbundle By Name(w2947) -> ("Image"=w2946:path)
                          "Image Path" <- w2946
                          n1367 = control-ref of="OperPict"() -> (w2950:refnum<vi>)
                          n1368 = call <vilib>:"Graphics.Read Image File and Auto Scale for 2D Picture.vi"("2D Pict Ref"=w2950, "File"=w2946) -> ("error out"=w2948:errorcluster, "Zoom Factor"=w2942:dbl, "2D Pict"=→"OperPict":picture)  [unwired: 7 in]
                          n1369 = property on="Status" class="Str"("Text.Text"="Waiting for Operator input on Image page.", "Text.BGColor"=u32 16774001, "Blinking"=TRUE) -> ()  [unwired: 2 in, 2 out]
                          n1370 = local write "Zoom Img"(w2942) -> ()
                        }
                        frame "Get Input" {
                          w2953 = T6."Image1" ("Test Status Tab")
                          w2963 = 300.0
                          n1371 = property on="OperOK" class="Bool"("Key Focus"=TRUE) -> ()  [unwired: 2 in, 2 out]
                          n1372 = Multiply(x=w2963, y=1000.0) -> (x*y=w2965:dbl)
                          n1373 = Tick Count (ms)() -> (millisecond timer value=w2962:u32)
                          n1374 = To Unsigned Long Integer(number=w2965) -> (unsigned 32bit integer=w2961:u32)
                          n1375 = while {
                            tunnel: w2962 -> [w2981]
                            tunnel: [w2975] -> w2955
                            tunnel: ["OperOK"] -> w2956
                            tunnel: w2961 -> [w2970]
                            stop <- w2983 stop-if-true
                            # "Wait for input"
                            n1376 = Tick Count (ms)() -> (millisecond timer value=w2982:u32)
                            n1377 = local read "Abort Flag"() -> (w2984:bool)
                            n1378 = Subtract(x=w2982, y=w2981) -> (x-y=w2969:u32)
                            n1379 = Subtract(x=w2970, y=w2969) -> (x-y=w2968:u32)
                            n1380 = Greater?(x=w2969, y=w2970) -> (0:w2976:bool)
                            n1381 = And(x=w2976, y="TO_En") -> (x .and. y?=w2975:bool)
                            n1382 = To Double Precision Float(number=w2968) -> (double precision float=w2979:dbl)
                            n1383 = Wait (ms)(milliseconds to wait=u32 100) -> ()  [unwired: 1 out]
                            n1384 = Divide(x=w2979, y=1000.0) -> (x/y=w2972:dbl)
                            n1385 = Greater Or Equal To 0?(x=w2972) -> (x >= 0?=w2973:bool)
                            n1386 = Compound Arithmetic op=OR(w2975, "OperOK", "OperNo", w2984) -> (w2983:bool)
                            n1387 = Select(t=w2972, s=w2973, f=0.0) -> (s? t:f=w2974:dbl)
                            n1388 = local write "OperCntDwn"(w2974) -> ()
                          }
                          n1389 = local write "Test Status Tab"(w2953) -> ()
                          n1390 = local write "Test Status Tab Sel"(w2953) -> ()
                          n1391 = case shown="False" w2955 {
                            tunnel: [_ errorcluster {"status"=TRUE, "code"=-2, "source"="Operator did not respond to image inspection prompt within timeout interval."} ("error constant")] -> w2954
                            frame False {
                            }
                            frame True {
                            }
                          }
                          n1392 = Bundle By Name(cluster=w2959, "Timeout"=w2955, "OK"=w2956) -> (w2958:T79)
                          "OperCntDwn" <- w2963
                        }
                        frame "Done", Default {
                          w2988 = T36."Disabled and Grayed Out" ("Disabled")
                          n1393 = Unbundle By Name(w2999) -> ("OK"=w3000:bool)
                          n1394 = Unbundle By Name(w2999) -> ("Name"=w2998:string)
                          n1395 = Unbundle By Name(w3014) -> ("Opts.DispDetails"=w3012:bool)
                          n1396 = Not(x=w3000) -> (.not. x?=w2990:bool)
                          n1397 = Select(t="PASS" ("Category"), s=w3000, f="FAIL" ("Category")) -> (s? t:f=w3009:string)
                          n1398 = Select(t=1, s=w3012, f=0) -> (s? t:f=w2987:i32)
                          n1399 = call "Result.Build Attribute Result Item.ctl"("ForceFail"=w2990, "Log(F)/Pass(T)"=TRUE, "Error In(Result Error)"=w3001, "Value"=w3009, "Name"=w2998, "Category"="Oper Prompt") -> ("Attribute"=w2997:T43)  [unwired: 3 in, 2 out]
                          n1400 = local write "Test Status Tab"(w2987) -> ()
                          n1401 = local write "Test Status Tab Sel"(w2987) -> ()
                          n1402 = property on="OperOK" class="Bool"("Key Focus"=FALSE, "DisabledEnum"=w2988) -> ()  [unwired: 2 in, 2 out]
                          n1403 = Build Array(w2997) -> (w3004:T43[])
                          n1404 = property on="OperNo" class="Bool"("DisabledEnum"=w2988) -> ()  [unwired: 2 in, 2 out]
                          n1405 = Select(t="Image Check: PASS" ("Category"), s=w2990, f="Image Check: FAIL" ("Category")) -> (s? t:f=w2995:string)
                          n1406 = To Variant(anything=w3004) -> (Variant=w3003:variant)
                          n1407 = call <vilib>:"Q.Enqueue Task.vi"("Top of Q"=TRUE, "Data1"=w3003, "Task Name"="Result - Attributes", "Q In"=w2996) -> ()  [unwired: 6 in, 2 out]
                          n1408 = property on="Open Image File" class="Bool"("DisabledEnum"=w2988) -> ()  [unwired: 2 in, 2 out]
                          n1409 = property on="Status" class="Str"("Text.Text"=w2995, "Text.BGColor"=u32 13816530, "Blinking"=FALSE) -> ()  [unwired: 2 in, 2 out]
                        }
                      }
                      n1410 = case shown="Error" w2901 {
                        tunnel: [w2910 "Done"] -> w2900
                        tunnel: w2899 -> [w2910 _]
                        frame No Error {
                        }
                        frame Error {
                        }
                      }
                    }
                  }
                  frame "Int" {
                    n1411 = Index Array(array=w3033) -> (element=w3032:string)  [unwired: 1 in]
                    n1412 = Fract/Exp String To Number(string=w3032) -> (number=w3031:dbl)  [unwired: 3 in, 1 out]
                    n1413 = Quotient & Remainder(x=w3031, y=1.0) -> (x-y*floor(x/y)=w3021:dbl, floor(x/y)=w3024:dbl)
                    n1414 = To Long Integer(number=w3024) -> (32bit integer=w3023:i32)
                    n1415 = Number To Decimal String(number=w3023) -> (decimal integer string=w3022:string)  [unwired: 1 in]
                    n1416 = Number To Fractional String(number=w3021) -> (F-format string=w3018:string)  [unwired: 3 in]
                    n1417 = Build Array("FractValue", w3018) -> (w3027:string[])
                    n1418 = Build Array("IntValue", w3022) -> (w3017:string[])
                    n1419 = Unbundle By Name(w3026) -> ("SeqMgr"=w3030:refnum<class "SeqMgr.lvclass">)
                    n1420 = Build Array(w3027, w3017) -> (w3028:string[][])
                    n1421 = call <vilib>:"SeqMgr.Variables - Add, Replace.vi"("Name, Value"=w3028, "SeqMgr in"=w3030) -> ("SeqMgr out"=w3029:refnum<class "SeqMgr.lvclass">)  [unwired: 8 in, 1 out]
                    n1422 = Bundle By Name(cluster=w3026, "SeqMgr"=w3029) -> (w3025:T73)
                  }
                  frame "ImagePromptLeftRight" {
                    # "ImagePromptLeftRight(PromptMessage,ImageFilePathLeft, ImageFilePathRight, Zoom,[ResultAttributeName, ResultAttributeCategory])"
                    n1423 = while {
                      shift-right: [w3044] -> _
                      shift-left: "Init" -> [w3048]
                      shift-right: [w3046] -> _
                      shift-left: _ -> [w3047]
                      tunnel: w3037 -> [w3045]
                      shift-right: [w3041] -> _
                      shift-left: _ -> [w3042]
                      tunnel: w3035 -> [w3040]
                      tunnel: w3036 -> [w3039]
                      stop <- w3043 stop-if-true
                      n1424 = case shown="\"Done\", Default" w3048 {
                        tunnel: w3047 -> [_ w3087 w3122 w3155 w3183 w3195]
                        tunnel: [w3058 w3092 w3121 w3154 w3183 w3195] -> w3046
                        tunnel: w3045 -> [w3072 _ _ _ _ _]
                        tunnel: ["File Check" w3088 w3120 w3153 "Done" "Done"] -> w3044
                        tunnel: [_ _ _ _ _ TRUE] -> w3043
                        tunnel: w3042 -> [_ _ _ _ _ w3203]
                        tunnel: [errorcluster {"status"=FALSE, "code"=0, "source"=""} ("error constant") _ _ _ _ w3203] -> w3041
                        tunnel: w3040 -> [_ _ _ _ _ w3190]
                        tunnel: w3039 -> [_ _ _ _ w3184 _]
                        frame "Init" {
                          w3053 = 1.0  # Zoom
                          w3060 = FALSE  # OK
                          w3049 = T6."Image2" ("Test Status Tab")
                          w3061 = picture data[5B] ("Rigth Image")
                          w3068 = T43 {"Cnt"=0, "Step"="", "Category"="", "Name"="", "Value"="", "Status"=0, "Code"=0, "Desc"="", "Time"=timestamp(0 s since 1904-01-01)}  # Result
                          w3077 = path ""  # Right
                          w3078 = path ""  # Left
                          n1425 = Index Array(array=w3072) -> (element #1=w3070:string, element #2=w3067:string, element #3=w3066:string, element #4=w3055:string, element #5=w3056:string, element #6=w3057:string)  [unwired: 6 in]
                          n1426 = Format Into String(format string="Operator input required: %s.", w3070) -> (resulting string=w3069:string)  [unwired: 2 in, 1 out]
                          n1427 = Fract/Exp String To Number(string=w3055) -> (number=w3054:dbl)  [unwired: 3 in, 1 out]
                          n1428 = String To Path(string=w3067) -> (path=w3063:path)
                          n1429 = String To Path(string=w3066) -> (path=w3062:path)
                          n1430 = property on="Status" class="Str"("Text.Text"=w3069, "Text.BGColor"=u32 16774001, "Blinking"=TRUE) -> ()  [unwired: 2 in, 2 out]
                          n1431 = local write "Test Status Tab"(w3049) -> ()
                          n1432 = local write "Test Status Tab Sel"(w3049) -> ()
                          n1433 = In Range and Coerce(upper limit=1.0, x=w3054, lower limit=0.1 ("upper limit")) -> (coerced(x)=w3050:dbl)  [unwired: 1 out]
                          n1434 = case shown="\"\"" w3057 {
                            selector: w3057 -> [w3079 _]
                            tunnel: [w3079 "Prompt"] -> w3064
                            frame Default {
                            }
                            frame "" {
                            }
                          }
                          n1435 = case shown="\"\"" w3056 {
                            selector: w3056 -> [w3081 _]
                            tunnel: [w3081 "Image Prompt"] -> w3065
                            frame Default {
                            }
                            frame "" {
                            }
                          }
                          n1436 = Bundle("Left"=w3078, "Right"=w3077, "Result"=w3068, "OK"=w3060, "Zoom"=w3053) -> (w3059:T80)  [unwired: 1 in]
                          n1437 = Bundle By Name(cluster=w3059, "Zoom"=w3050, "Left"=w3063, "Right"=w3062, "Result.Name"=w3065, "Result.Category"=w3064) -> (w3058:T80)
                          n1438 = local write "Zoom Right"(w3050) -> ()
                          n1439 = local write "Zoom Left"(w3050) -> ()
                          n1440 = local write "Rigth Image"(w3061) -> ()
                          n1441 = local write "Left Image"(w3061) -> ()
                        }
                        frame "File Check" {
                          n1442 = Unbundle By Name(w3087) -> ("Left"=w3086:path, "Right"=w3085:path)
                          n1443 = call <vilib>:"File.Check if File or Folder Exists.vi"("Path"=w3085) -> ("Exists"=w3084:bool, "Dup Path"=w3090:path)  [unwired: 6 in, 3 out]
                          n1444 = call <vilib>:"File.Check if File or Folder Exists.vi"("Path"=w3086) -> ("Exists"=w3083:bool, "Dup Path"=w3091:path)  [unwired: 6 in, 3 out]
                          n1445 = And(x=w3083, y=w3084) -> (x .and. y?=w3089:bool)
                          n1446 = case shown="False" w3089 {
                            tunnel: w3087 -> [w3103 w3112]
                            tunnel: [w3102 w3112] -> w3092
                            tunnel: w3091 -> [_ _]
                            tunnel: w3090 -> [_ _]
                            tunnel: ["Result" "Load Images"] -> w3088
                            tunnel: w3084 -> [w3096 _]
                            tunnel: w3083 -> [w3097 _]
                            frame False {
                              w3100 = T74 -5200 items=["No Error"=0, "Abort"=-2, "Misc"=-5000, "Fixture Error"=-5100, "File IO - General"=-5200, "FIle IO - Config Error"=-5201, "Instrument - General"=-5300, "Instrument - Serial Com"=-5301, "Instrument - Camera"=-5302, "Instrument - PS"=-5303, "Instrument - Oscilloscope"=-5304, "Instrument - Function Gen"=-5305, "Instrument - Load"=-5306, "Instrument - Meter"=-5307, "Instrument - Power Control"=-5308, "Instrument - Motion"=-5309, "Instrument - RF"=-5310, "System Exe"=-5400, "Image Processing"=-5500, "Communication"=-5600, "Script - Syntax Error"=-6000, "Script - Invalid Name or Param"=-6100, "Script - Timeout"=-6200, "Invalid Data"=-6300, "FW Update Error"=-6500] ("Std Code")
                              w3101 = T39 3 items=["LOG", "PASS", "FAIL", "ERROR"] ("Result.Status")
                              n1447 = case shown="True" w3097 {
                                tunnel: w3096 -> [w3106 w3110]
                                tunnel: [w3105 w3109] -> w3094
                                frame False {
                                n1448 = case shown="False" w3106 {
                                tunnel: ["Both left and right files do not exist." "Left file does not exist."] -> w3105
                                frame False {
                                }
                                frame True {
                                }
                                }
                                }
                                frame True {
                                n1449 = case shown="True" w3110 {
                                tunnel: ["Right file does not exist." _] -> w3109
                                frame False {
                                }
                                frame True {
                                # "Will not get here"
                                }
                                }
                                }
                              }
                              n1450 = To Long Integer(number=w3100) -> (32bit integer=w3099:T74)
                              n1451 = Concatenate Strings("Image prompt error.  ", w3094) -> (w3095:string)
                              n1452 = Bundle By Name(cluster=w3103, "Result.Value"="Missing File", "Result.Status"=w3101, "Result.Code"=w3099, "Result.Desc"=w3095) -> (w3102:T80)
                            }
                            frame True {
                            }
                          }
                        }
                        frame "Load Images" {
                          n1453 = Unbundle By Name(w3122) -> ("Left"=w3126:path, "Right"=w3125:path, "Zoom"=w3114:dbl)
